vi "RefMem PtByPt RT Driver VI (Inline).vi"(7 "Operation":T1, 11 "Device Reference in":T2 format="%.0x") -> (0 "Error Code":i32)   [LabVIEW 2010, in "RefMem PtByPt Custom Device.lvlib"]
uses:
  RefMem PtByPt Custom Device.lvlib
  <vilib>/NI Veristand/Custom Device API/Custom Device Item Ref.ctl
  <vilib>/NI VeriStand/Custom Device API/Hardware Interface Driver VI Operation.ctl
  Controls/Inline RT Data Cluster.ctl
  Controls/RT Chan Cluster.ctl
  <vilib>/NI Veristand/Custom Device API/Block Data Reference.ctl
  <vilib>/NI Veristand/Custom Device API/Data Reference.ctl
  Controls/Data Channel Type.ctl
  <vilib>/NI Veristand/Custom Device API/Data Access Type.ctl
  Controls/Global.vi
  <vilib>/NI Veristand/Custom Device API/Get Item Property (String).vi
  <vilib>/NI Veristand/Custom Device API/Custom Device API.lvlib
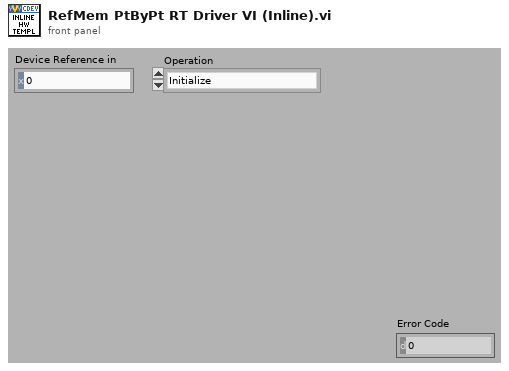
[diagram p1: front panel]
types:
  T1 = typedef "Custom Device API.lvlib/Hardware Interface Driver VI Operation.ctl" = enum16{"Initialize", "Start", "Read Data from HW", "Write Data to HW", "Close"}
  T2 = typedef "Custom Device API.lvlib/Custom Device Item Ref.ctl" = u64
  T3 = typedef "RefMem PtByPt Custom Device.lvlib/Inline RT Data Cluster.ctl" = cluster{"Read Chns":T4, "Write Chns":T4, "Stat Chns":cluster{"BD Refs":T5[], "Values":dbl[]}, "VISA res":refnum<visa-resource-name>}
  T4 = typedef "RefMem PtByPt Custom Device.lvlib/RT Chan Cluster.ctl" = cluster{"BD Refs":T5[], "Values":dbl[], "Adds":u32[]}
  T5 = typedef "Custom Device API.lvlib/Block Data Reference.ctl" = cluster{"Data Reference":T6, "Offset":i32, "Length":i32}
  T6 = typedef "Custom Device API.lvlib/Data Reference.ctl" = i32
  T7 = typedef "RefMem PtByPt Custom Device.lvlib/Data Channel Type.ctl" = enum16{"Read", "Write"}
  T8 = typedef "Custom Device API.lvlib/Data Access Type.ctl" = enum16{"Read", "Write"}
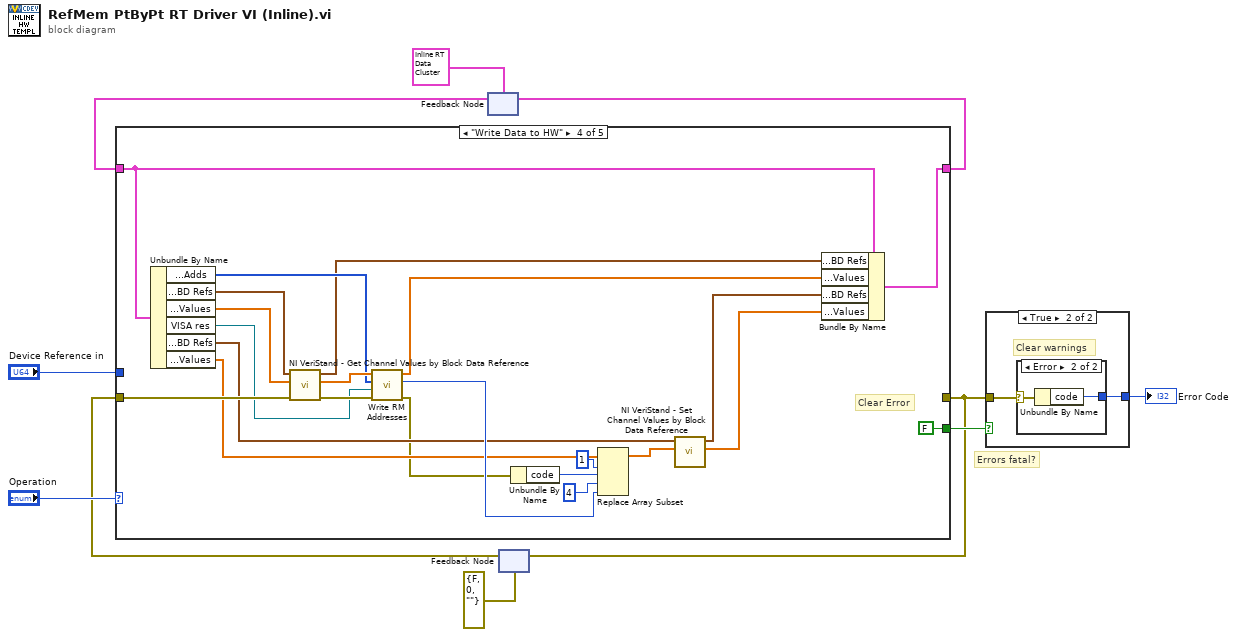
[diagram p0: block diagram]
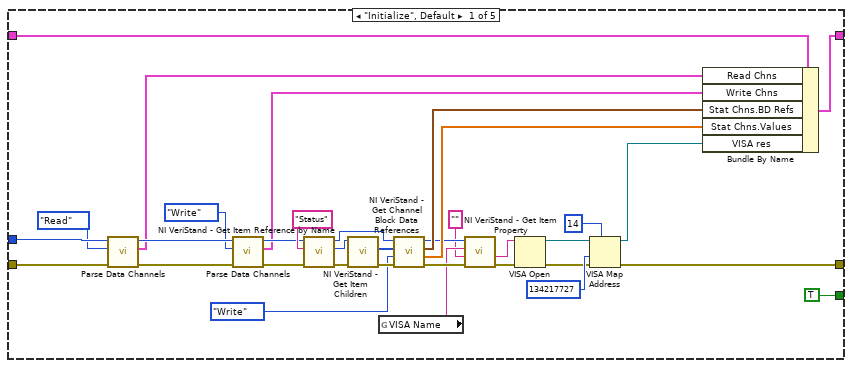
[diagram p4: hidden frame]
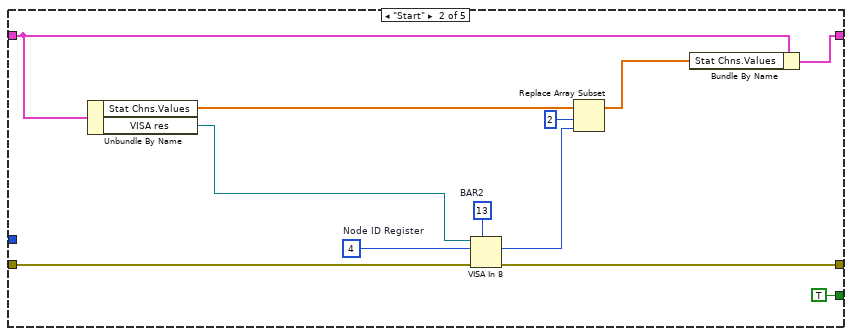
[diagram p5: hidden frame]
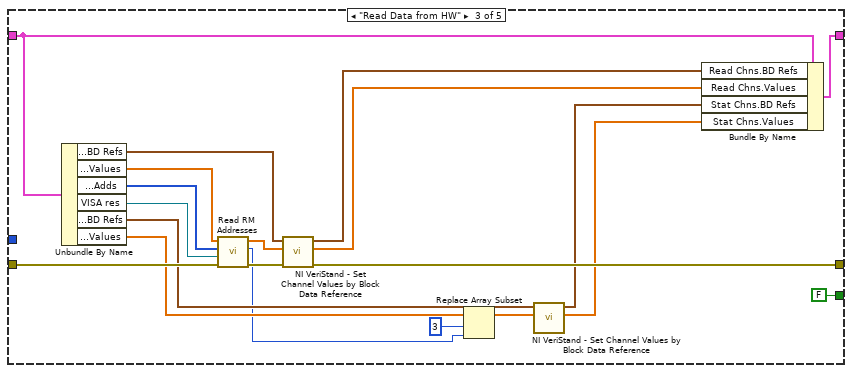
[diagram p6: hidden frame]
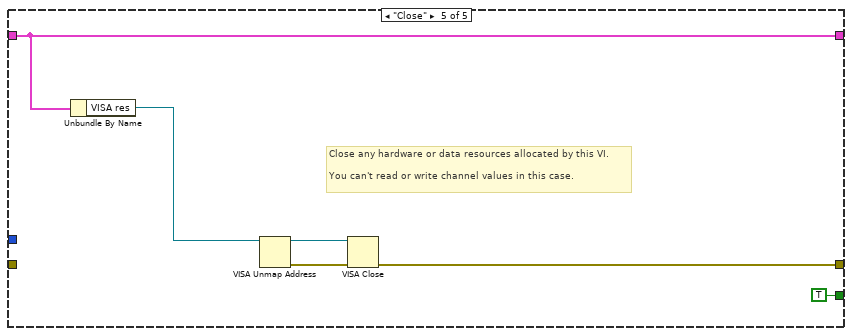
[diagram p7: hidden frame]
diagram:
  # "Errors fatal?"
  n1 = feedback #1(T3 {"Read Chns"={"BD Refs"=[], "Values"=[], "Adds"=[]}, "Write Chns"={"BD Refs"=[], "Values"=[], "Adds"=[]}, "Stat Chns"={"BD Refs"=[], "Values"=[]}, "VISA res"=""} ("RT Data")) -> (w1:T3)
  n2 = feedback #2(errorcluster {"status"=FALSE, "code"=0, "source"=""} ("error out")) -> (w3:errorcluster)
  n3 = case shown="\"Write Data to HW\"" "Operation" {
    tunnel: [w35 w50 w68 w89 w104] -> w9
    tunnel: w1 -> [w43 w51 w69 w90 w104]
    tunnel: "Device Reference in" -> [w44 _ _ _ _]
    tunnel: [TRUE TRUE FALSE FALSE TRUE] -> w6
    tunnel: [w24 w45 w64 _ w100] -> w4
    tunnel: w3 -> [w31 w53 w76 w97 _]
    frame "Initialize", Default {
      n4 = call "Parse Data Channels.vi"("error in"=w31, "DataChan Type"=Data_Channel_Type."Read", "Device Reference in"=w44) -> ("error out"=w18:errorcluster, "Channels"=w12:T4, "Device Reference out"=w17:T2)  [unwired: 6 in]
      n5 = call "Parse Data Channels.vi"("error in"=w18, "DataChan Type"=Data_Channel_Type."Write", "Device Reference in"=w17) -> ("error out"=w15:errorcluster, "Channels"=w11:T4, "Device Reference out"=w16:T2)  [unwired: 6 in]
      n6 = call <vilib>:"NI VeriStand - Get Item Reference by Name.vi"("error in (no error)"=w15, "Item Name"="Status", "Parent Ref in"=w16) -> ("error out"=w41:errorcluster, "Item Ref"=w40:T2, "Parent Ref out"=w36:T2)  [unwired: 5 in, 1 out]
      n7 = call <vilib>:"NI VeriStand - Get Item Children.vi"("error in (no error)"=w41, "Item Ref in"=w40) -> ("error out"=w39:errorcluster, "Child Refs"=w38:T2[])  [unwired: 6 in, 2 out]
      n8 = global read "Global.vi" "VISA Name"() -> (w28:string)
      n9 = call <vilib>:"NI VeriStand - Get Channel Block Data References.vi"("error in (no error)"=w39, "Access"=Data_Access_Type."Write", "Channel Refs"=w38, "Device Ref in"=w36) -> ("error out"=w30:errorcluster, "Values Array"=w33:dbl[], "Block Data Refs"=w34:T5[], "Device Ref out"=w29:T2)  [unwired: 4 in]
      n10 = call-poly <vilib>:"NI VeriStand - Get Item Property.vi"("error in (no error)"=w30, "Default Value"="", "Property Name"=w28, "Item Ref in"=w29) -> ("error out"=w22:errorcluster, "Value"=w21:string)  [unwired: 4 in, 2 out]
      n11 = VISA Open(error in (no error)=w22, VISA resource name=w21) -> (VISA resource name=w20:refnum<visa-resource-name>, error out=w23:errorcluster)  [unwired: 3 out]
      n12 = VISA Map Address(7:u16 14 ("BAR3"), 8:w23, 9:u32 134217727 ("map size (0)"), 11:w20) -> (0:w24:errorcluster, 3:w19:refnum<visa-resource-name>)  [unwired: 2 in]
      n13 = Bundle By Name(cluster=w43, "Read Chns"=w12, "Write Chns"=w11, "Stat Chns.BD Refs"=w34, "Stat Chns.Values"=w33, "VISA res"=w19) -> (w35:T3)
    }
    frame "Start" {
      w55 = u32 4  # Node ID Register
      w54 = u16 13  # BAR2
      n14 = Unbundle By Name(w51) -> ("Stat Chns.Values"=w49:dbl[], "VISA res"=w52:refnum<visa-resource-name>)
      n15 = VISA In 8(7:w54, 8:w53, 10:w55, 11:w52) -> (0:w45:errorcluster, 2:w46:u8)  [unwired: 1 out]
      n16 = Replace Array Subset(array=w49, new element=w46, index=2) -> (w48:dbl[])
      n17 = Bundle By Name(cluster=w51, "Stat Chns.Values"=w48) -> (w50:T3)
    }
    frame "Read Data from HW" {
      n18 = Unbundle By Name(w69) -> ("Read Chns.BD Refs"=w73:T5[], "Read Chns.Values"=w71:dbl[], "Read Chns.Adds"=w70:u32[], "VISA res"=w59:refnum<visa-resource-name>, "Stat Chns.BD Refs"=w65:T5[], "Stat Chns.Values"=w63:dbl[])
      n19 = call "Read RM Addresses.vi"("error in"=w76, "Session"=w59, "Addresses"=w70, "Old Values"=w71) -> ("error out"=w75:errorcluster, "Read Duration"=w57:u32, "Updated Values"=w72:dbl[])  [unwired: 5 in]
      n20 = call <vilib>:"NI VeriStand - Set Channel Values by Block Data Reference.vi"("error in (no error)"=w75, "Values Array in"=w72, "Block Data Ref"=w73) -> ("error out"=w64:errorcluster, "Values Array out"=w66:dbl[], "Block Data Ref dup"=w67:T5[])  [unwired: 6 in]
      n21 = Replace Array Subset(array=w63, new element=w57, index=3) -> (w62:dbl[])
      n22 = call <vilib>:"NI VeriStand - Set Channel Values by Block Data Reference.vi"("Values Array in"=w62, "Block Data Ref"=w65) -> ("Values Array out"=w60:dbl[], "Block Data Ref dup"=w61:T5[])  [unwired: 7 in, 1 out]
      n23 = Bundle By Name(cluster=w69, "Read Chns.BD Refs"=w67, "Read Chns.Values"=w66, "Stat Chns.BD Refs"=w61, "Stat Chns.Values"=w60) -> (w68:T3)
    }
    frame "Write Data to HW" {
      # "Clear Error"
      n24 = Unbundle By Name(w90) -> ("Write Chns.Adds"=w91:u32[], "Write Chns.BD Refs"=w96:T5[], "Write Chns.Values"=w95:dbl[], "VISA res"=w93:refnum<visa-resource-name>, "Stat Chns.BD Refs"=w82:T5[], "Stat Chns.Values"=w81:dbl[])
      n25 = call <vilib>:"NI VeriStand - Get Channel Values by Block Data Reference.vi"("error in (no error)"=w97, "Values Array in"=w95, "Block Data Ref"=w96) -> ("error out"=w94:errorcluster, "Values Array out"=w92:dbl[], "Block Data Ref dup"=w78:T5[])  [unwired: 6 in]
      n26 = call "Write RM Addresses.vi"("error in"=w94, "Session"=w93, "Addresses"=w91, "Values"=w92) -> ("error out"=w79:errorcluster, "Write Duration"=w84:u32, "Values"=w88:dbl[])  [unwired: 5 in]
      n27 = Unbundle By Name(w79) -> ("code"=w86:i32)
      n28 = Replace Array Subset(array=w81, new element #1=w86, index #1=1 ("index"), new element #2=w84, index #2=4 ("index")) -> (w83:dbl[])
      n29 = call <vilib>:"NI VeriStand - Set Channel Values by Block Data Reference.vi"("Values Array in"=w83, "Block Data Ref"=w82) -> ("Values Array out"=w80:dbl[], "Block Data Ref dup"=w77:T5[])  [unwired: 7 in, 1 out]
      n30 = Bundle By Name(cluster=w90, "Write Chns.BD Refs"=w78, "Write Chns.Values"=w88, "Stat Chns.BD Refs"=w77, "Stat Chns.Values"=w80) -> (w89:T3)
    }
    frame "Close" {
      # "Close any hardware or data resources allocated by this VI.\n\nYou can't read or write channel values in this case."
      n31 = Unbundle By Name(w104) -> ("VISA res"=w102:refnum<visa-resource-name>)
      n32 = VISA Unmap Address(11:w102) -> (0:w101:errorcluster, 3:w99:refnum<visa-resource-name>)  [unwired: 1 in]
      n33 = VISA Close(VISA resource name=w99, error in (no error)=w101) -> (error out=w100:errorcluster)
    }
  }
  n34 = feedback-in #1(w9) -> ()
  n35 = feedback-in #2(w4) -> ()
  n36 = case shown="True" w6 {
    tunnel: w4 -> [_ w106]
    tunnel: [_ w105] -> w5
    frame False {
    }
    frame True {
      # "Clear warnings"
      n37 = case shown="Error" w106 {
        selector: w106 -> [_ w108]
        tunnel: [_ w107] -> w105
        frame No Error {
        }
        frame Error {
          n38 = Unbundle By Name(w108) -> ("code"=w107:i32)
        }
      }
    }
  }
  "Error Code" <- w5
